vi "Hanning Filter.vi"(10 "Input 2":dbl, 11 "Input":dbl) -> (2 "Filtered2":dbl, 3 "Filtered":dbl)   [LabVIEW 2013, in "main.lvlib"]
uses:
  main.lvlib
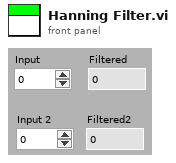
[diagram p1: front panel]
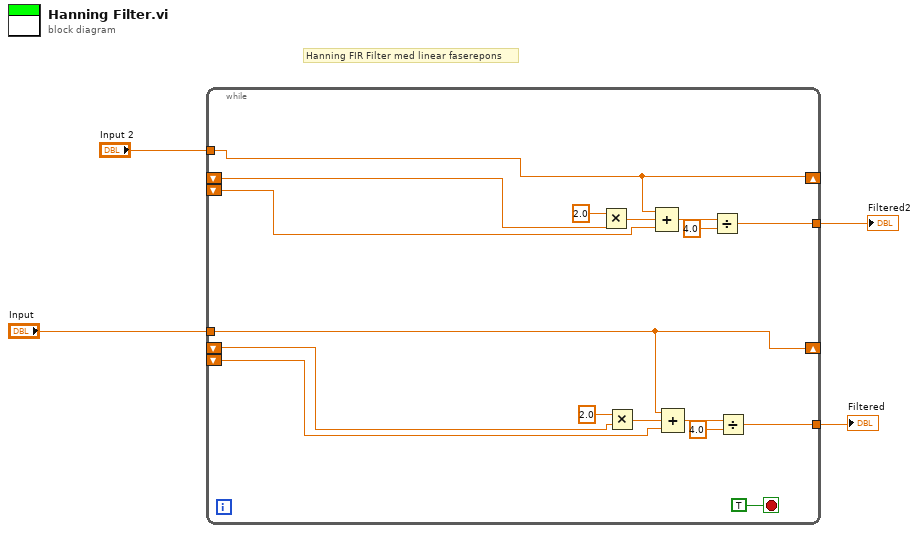
[diagram p0: block diagram]
diagram:
  # "Hanning FIR Filter med linear faserepons"
  n1 = while {
    shift-right: [w20] -> _
    shift-left: _ -> [w21]
    tunnel: "Input" -> [w20]
    tunnel: [w18] -> w3
    shift-left: _ -> [w17]
    shift-right: [w16] -> _
    shift-left: _ -> [w15]
    tunnel: "Input 2" -> [w16]
    shift-left: _ -> [w14]
    tunnel: [w13] -> w1
    stop <- TRUE stop-if-true
    n2 = Multiply(x=2.0, y=w15) -> (x*y=w7:dbl)
    n3 = Multiply(x=2.0, y=w21) -> (x*y=w11:dbl)
    n4 = Compound Arithmetic op=ADD(w16, w7, w14) -> (w6:dbl)
    n5 = Compound Arithmetic op=ADD(w20, w11, w17) -> (w10:dbl)
    n6 = Divide(x=w6, y=4.0) -> (x/y=w13:dbl)
    n7 = Divide(x=w10, y=4.0) -> (x/y=w18:dbl)
  }
  "Filtered" <- w3
  "Filtered2" <- w1
